vi "Chain.vi"(6 "Events":T1, 7 "Action":T2, 8 "error in (no error)":errorcluster, 9 "Parent":string, 10 "Panel":string) -> (0 "error out":errorcluster, 1 "Event Lookup":variant, 2 "Full Chain":variant)   [LabVIEW 2020, in "Panel.lvlib" / "Panel Registry.lvclass"]
doc: "Functional Global to store info about the panel chain.\n----\nCopyright: MGI 2017\nAuthor: Derek Trepanier"
uses:
  <vilib>/MGI/Panel Manager/Panel/Panel Registry/Panel Registry.lvclass
  <vilib>/MGI/Panel Manager/Panel/Cursor/Cursor.lvclass
  <vilib>/MGI/Panel Manager/Panel/Cursor/Lookup Actions.ctl
  <vilib>/MGI/Panel Manager/Panel/Panel Registry/Chain Action.ctl
  <vilib>/MGI/Panel Manager/Panel/Panel Helper/Events.ctl
  <vilib>/MGI/Panel Manager/Panel/Panel Helper/Panel Helper.lvclass
  <vilib>/MGI/Panel Manager/Panel/Panel Helper/Panel Events.ctl
panel:
  out "Debug Tree":string(tree)
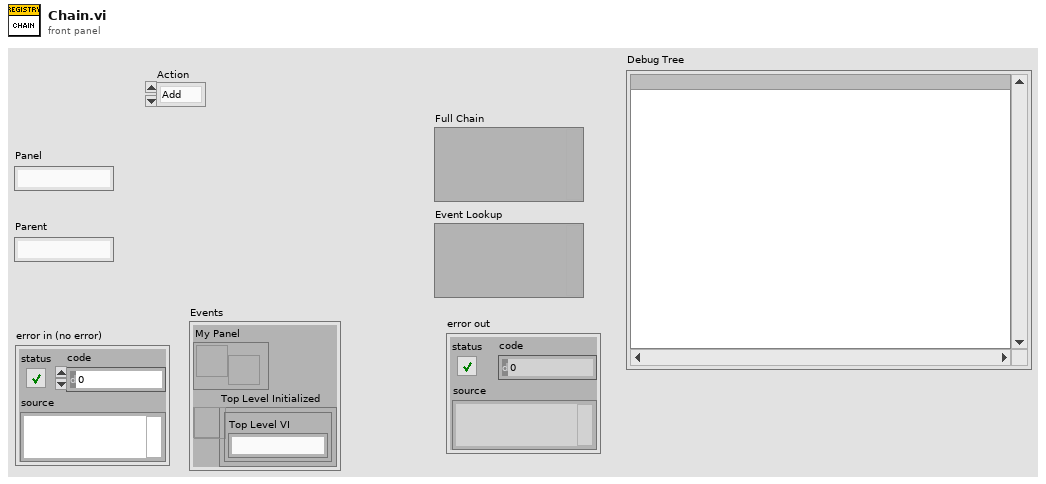
[diagram p1: front panel]
types:
  T1 = typedef "Panel.lvlib/Panel Helper.lvclass/Panel Events.ctl" = cluster{"My Panel":refnum<user-event>, "Top Level Initialized":refnum<user-event>}
  T2 = typedef "Chain Action.ctl" = enum16{"Add", "Read", "Remove"}
  T3 = typedef "Panel.lvlib/Cursor.lvclass/Lookup Actions.ctl" = enum16{"Init", "Get", "Destroy"}
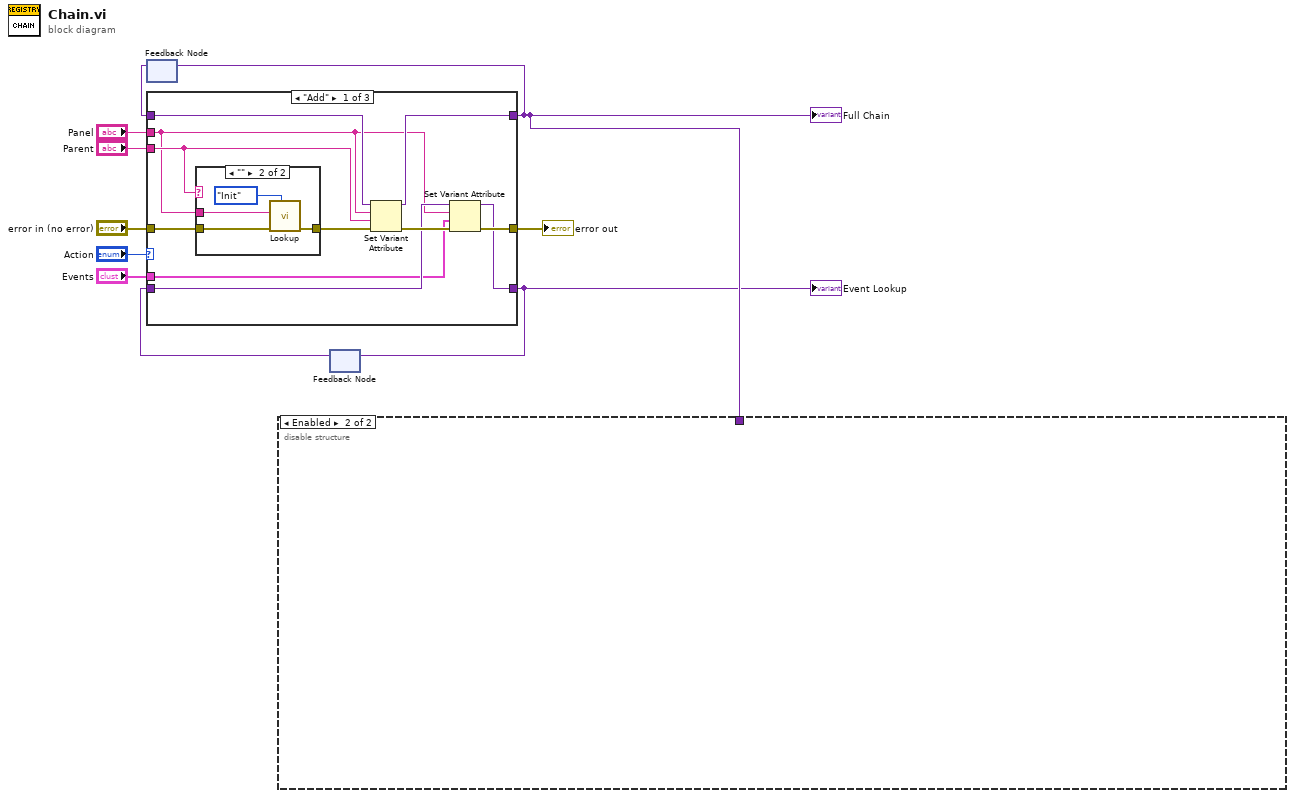
[diagram p0: block diagram]
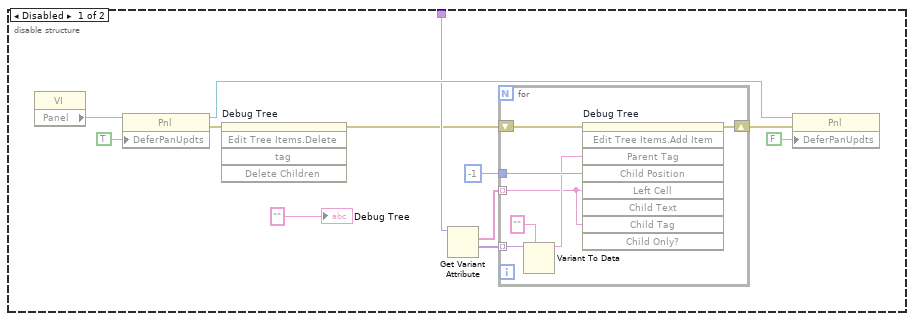
[diagram p2: hidden frame]
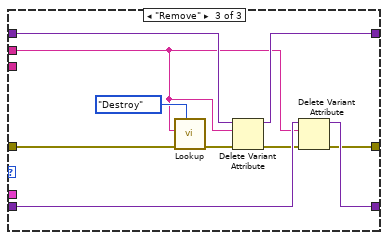
[diagram p5: hidden frame]
diagram:
  n1 = feedback #1() -> (w9:variant)  [unwired: 1 in]
  n2 = feedback #2() -> (w2:variant)  [unwired: 1 in]
  n3 = case shown="\"Add\"" "Action" {
    tunnel: "Panel" -> [w12 _ w30]
    tunnel: [w21 w29 w38] -> w4
    tunnel: w9 -> [w20 w29 w39]
    tunnel: "Parent" -> [w17 _ _]
    tunnel: [w15 w28 w31] -> w6
    tunnel: "error in (no error)" -> [w19 w28 w37]
    tunnel: [w14 w27 w33] -> w3
    tunnel: w2 -> [w13 w27 w34]
    tunnel: "Events" -> [w11 _ _]
    frame "Add" {
      n4 = case shown="\"\"" w17 {
        tunnel: w19 -> [w22 w26]
        tunnel: [w22 w23] -> w18
        tunnel: w12 -> [_ w25]
        frame Default {
        }
        frame "" {
          n5 = call <vilib>:"Lookup.vi"("Action"=Lookup_Actions."Init", "error in (no error)"=w26, "Top Level VI"=w25) -> ("error out"=w23:errorcluster)  [unwired: 7 in, 1 out]
        }
      }
      n6 = Set Variant Attribute(Variant=w20, name=w12, value=w17, error in=w18) -> (Variant out=w21:variant, error out=w16:errorcluster)  [unwired: 1 out]
      n7 = Set Variant Attribute(Variant=w13, name=w12, value=w11, error in=w16) -> (Variant out=w14:variant, error out=w15:errorcluster)  [unwired: 1 out]
    }
    frame "Read" {
    }
    frame "Remove" {
      n8 = call <vilib>:"Lookup.vi"("Action"=Lookup_Actions."Destroy", "error in (no error)"=w37, "Top Level VI"=w30) -> ("error out"=w36:errorcluster)  [unwired: 7 in, 1 out]
      n9 = Delete Variant Attribute(4:w36, 6:w30, 7:w39) -> (0:w32:errorcluster, 3:w38:variant)  [unwired: 1 out]
      n10 = Delete Variant Attribute(4:w32, 6:w30, 7:w34) -> (0:w31:errorcluster, 3:w33:variant)  [unwired: 1 out]
    }
  }
  "error out" <- w6
  "Full Chain" <- w4
  "Event Lookup" <- w3
  n11 = feedback-in #1(w4) -> ()
  n12 = disable-structure shown="Enabled" {
    disable-tunnel: w4 -> [w43 _]
    frame Disabled {
      n13 = property class="VI"() -> ("Panel"=w51:refnum<vi>)  [unwired: 2 in, 2 out]
      n14 = property class="Pnl"(reference=w51, "DeferPanUpdts"=TRUE ("Defer Panel Updates")) -> (reference out=w48:refnum<vi>, error out=w49:errorcluster)  [unwired: 1 in]
      n15 = invoke on="Debug Tree" class="Tree (strict)" method="Edit Tree Items.Delete"(error in=w49) -> (error out=w42:errorcluster)  [unwired: 4 in, 4 out]
      n16 = Get Variant Attribute(Variant=w43) -> (names=w45:string[], values=w44:variant[])  [unwired: 3 in, 2 out]
      n17 = for {
        tunnel: -1 ("Child Position") -> [w58]
        tunnel: w45 -> [w52] mode=indexing
        tunnel: w44 -> [w55] mode=indexing
        shift-right: [w56] -> w41
        shift-left: w42 -> [w57]
        n18 = Variant To Data(type="", Variant=w55) -> (data=w53:string)  [unwired: 1 in, 1 out]
        n19 = invoke on="Debug Tree" class="Tree (strict)" method="Edit Tree Items.Add Item"(error in=w57, "Parent Tag"=w53, "Child Position"=w58, "Left Cell"=w52, "Child Tag"=w52) -> (error out=w56:errorcluster)  [unwired: 4 in, 8 out]
      }
      n20 = property class="Pnl"(reference=w48, error in=w41, "DeferPanUpdts"=FALSE ("Defer Panel Updates")) -> ()  [unwired: 2 out]
      "Debug Tree" <- "" ("Debug Tree")
    }
    frame Enabled {
    }
  }
  n21 = feedback-in #2(w3) -> ()
